vi "SmartSEM Remote API FIB gun state.vi"(8 "error in":errorcluster, 11 "Api":refnum<k7>(container)) -> (0 "error out":errorcluster={"status"=FALSE, "code"=-2147417851, "source"=""}, 2 "FIB Gun State":string, 3 "Api out":refnum<k7>)   [LabVIEW 2018]
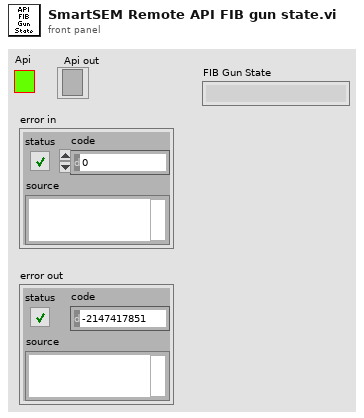
[diagram p1: front panel]
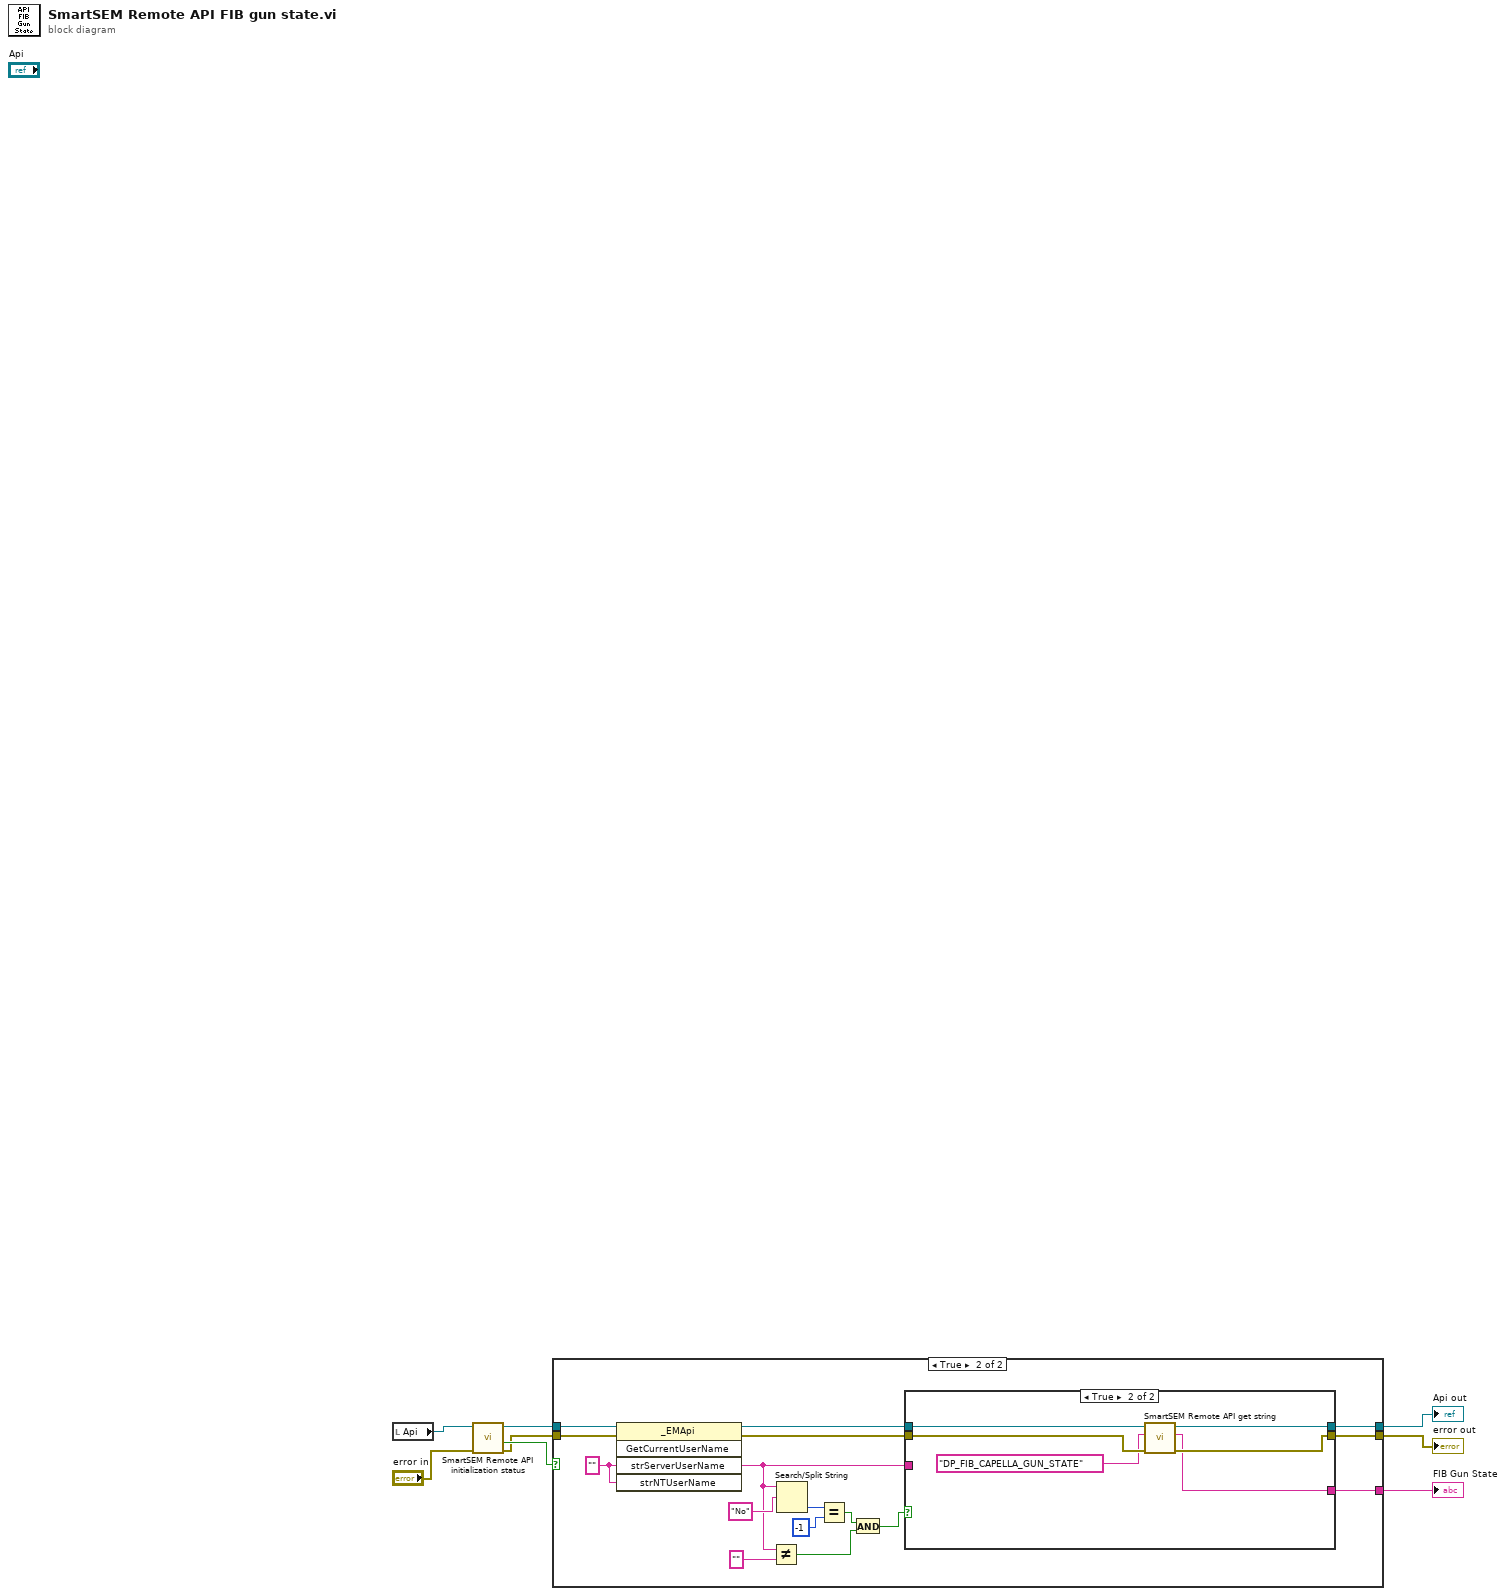
[diagram p0: block diagram]
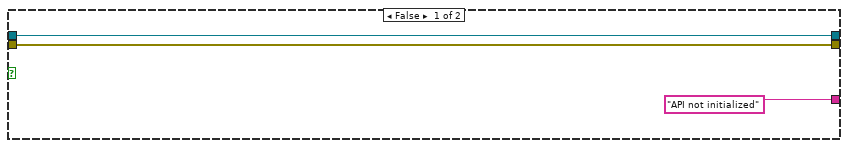
[diagram p2: hidden frame]
diagram:
  n1 = local read "Api"() -> (w5:refnum<k7>)
  n2 = call "SmartSEM Remote API initialization status.vi"("error in"="error in", "Api in"=w5) -> ("error out"=w2:errorcluster, "API initialized"=w3:bool, "Api out"=w1:refnum<k7>)  [unwired: 7 in]
  n3 = case shown="True" w3 {
    tunnel: w1 -> [w10 w18]
    tunnel: w2 -> [w9 w17]
    tunnel: [w10 w27] -> w8
    tunnel: [w9 w26] -> w7
    tunnel: ["API not initialized" ("lpszParam") w22] -> w6
    frame False {
    }
    frame True {
      w23 = "" ("strServerUserName")
      n4 = invoke class="_EMApi" method="GetCurrentUserName"(reference=w18, error in=w17, "strServerUserName"=w23, "strNTUserName"=w23) -> (reference out=w25:refnum<k7>, error out=w24:errorcluster, "strServerUserName"=w16:string)  [unwired: 1 in, 2 out]
      n5 = Not Equal?(x=w16, y="") -> (x != y?=w12:bool)
      n6 = Search/Split String(string=w16, search string/char (-)="No" ("strServerUserName")) -> (offset of match=w20:i32)  [unwired: 1 in, 2 out]
      n7 = Equal?(x=w20, y=-1) -> (x = y?=w14:bool)
      n8 = And(x=w14, y=w12) -> (x .and. y?=w13:bool)
      n9 = case shown="True" w13 {
        tunnel: [w30 w33] -> w27
        tunnel: [w29 w32] -> w26
        tunnel: w25 -> [w30 w36]
        tunnel: w24 -> [w29 w35]
        tunnel: [w28 w31] -> w22
        tunnel: w16 -> [w28 _]
        frame False {
        }
        frame True {
          n10 = call "SmartSEM Remote API get string.vi"("error in"=w35, "lpszParam"="DP_FIB_CAPELLA_GUN_STATE", "Api"=w36) -> ("error out"=w32:errorcluster, "data"=w31:string, "Api out"=w33:refnum<k7>)  [unwired: 6 in]
        }
      }
    }
  }
  "Api out" <- w8
  "error out" <- w7
  "FIB Gun State" <- w6
